vi "mod_VCO.vi"(0 "e(n)":dbl, 5 "gain (kf)":dbl, 7 "carrier frequency (normalized)":dbl, 9 "initial phase (degrees)":dbl, 11 "error in (no error)":errorcluster, 13 "reset ?(T)":bool=TRUE) -> (4 "theta(n)":dbl, 15 "error out":errorcluster)   [LabVIEW 2020, in "niAMT.lvlib"]
uses:
  <vilib>/addons/Modulation/niAMT.lvlib
panel:
  # "theta (n)-theta (n-1) = kf*e(n)+2*pi*fc*n"
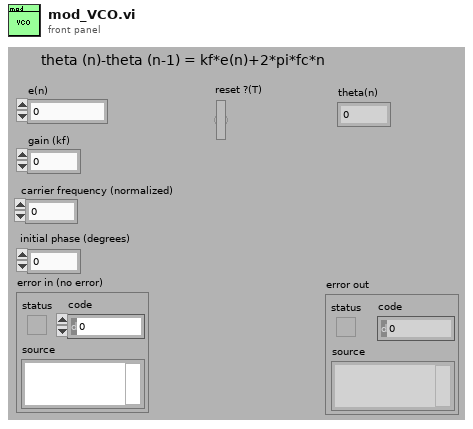
[diagram p1: front panel]
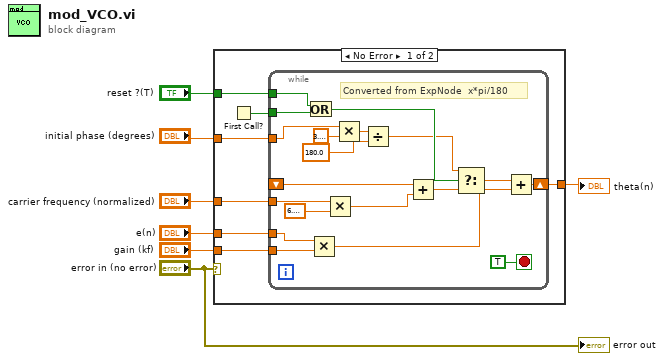
[diagram p0: block diagram]
diagram:
  n1 = case shown="No Error" "error in (no error)" {
    tunnel: "e(n)" -> [w14 _]
    tunnel: "gain (kf)" -> [w13 _]
    tunnel: "reset ?(T)" -> [w12 _]
    tunnel: "initial phase (degrees)" -> [w10 _]
    tunnel: "carrier frequency (normalized)" -> [w9 _]
    tunnel: [w8 _] -> w2
    frame No Error {
      n2 = First Call?() -> (First Call?: T/F=w11:bool)
      n3 = while {
        tunnel: w14 -> [w33]
        tunnel: w13 -> [w32]
        tunnel: w12 -> [w30]
        tunnel: w11 -> [w29]
        tunnel: w10 -> [w16]
        shift-right: [w24] -> w8
        shift-left: _ -> [w22]
        tunnel: w9 -> [w26]
        stop <- TRUE stop-if-true
        # "Converted from ExpNode\t\tx*pi/180"
        n4 = Or(x=w30, y=w29) -> (x .or. y?=w23:bool)
        n5 = Multiply(x=w33, y=w32) -> (x*y=w27:dbl)
        n6 = Multiply(x=w26, y=6.283185307179586) -> (x*y=w20:dbl)
        n7 = Multiply(x=w16, y=3.141592653589793) -> (x*y=w17:dbl)
        n8 = Divide(x=w17, y=180.0) -> (x/y=w15:dbl)
        n9 = Add(x=w22, y=w20) -> (x+y=w21:dbl)
        n10 = Select(t=w15, s=w23, f=w21) -> (s? t:f=w28:dbl)
        n11 = Add(x=w28, y=w27) -> (x+y=w24:dbl)
      }
    }
    frame Error {
    }
  }
  "theta(n)" <- w2
  "error out" <- "error in (no error)"
